vi "UnEscapeParser.vi"(1 "String In":string) -> (0 "String Out":string)   [LabVIEW 2020, in "DP_WebView.lvclass"]
uses:
  DP_WebView.lvclass
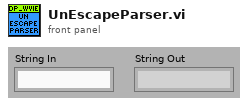
[diagram p1: front panel]
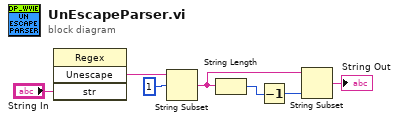
[diagram p0: block diagram]
diagram:
  n1 = invoke class="Regex" method="Unescape"("str"="String In") -> ("Unescape"=w3:string)  [unwired: 3 in, 3 out]
  n2 = String Subset(string=w3, offset (0)=1) -> (substring=w6:string)  [unwired: 1 in]
  n3 = String Length(string=w6) -> (length=w5:i32)
  n4 = Decrement(x=w5) -> (x-1=w4:i32)
  n5 = String Subset(string=w6, length (rest)=w4) -> (substring=→"String Out":string)  [unwired: 1 in]
